vi "M686_scanning.vi"(5 "notifier out":refnum<notifier>, 6 "Velocity":dbl, 8 "Axis":bool[](array[boolean]), 9 "Positions":dbl[](array[numeric]), 10 "Action":T1=enum."MVR", 11 "VISA resource name":refnum<visa-resource-name>) -> (0 "Special Function":string, 1 "Status":bool, 2 "Position Out":dbl[](array[numeric]))   [LabVIEW 2011]
uses:
  Controls/StageStates.ctl
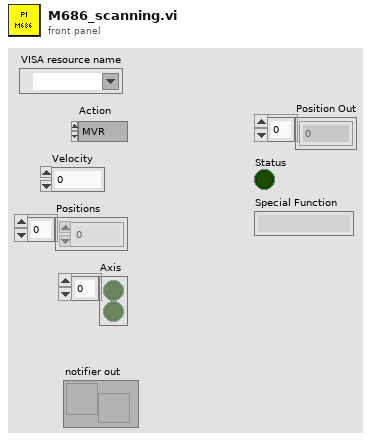
[diagram p1: front panel]
types:
  T1 = typedef "StageStates.ctl" = enum16{"POSITION", "MVR", "MOVE", "HALT", "ONTARGET", "ERROR", "EXIT", "HOME", "ZEROPOS", "NANOPOS", "QUIT", "ANALOG"}
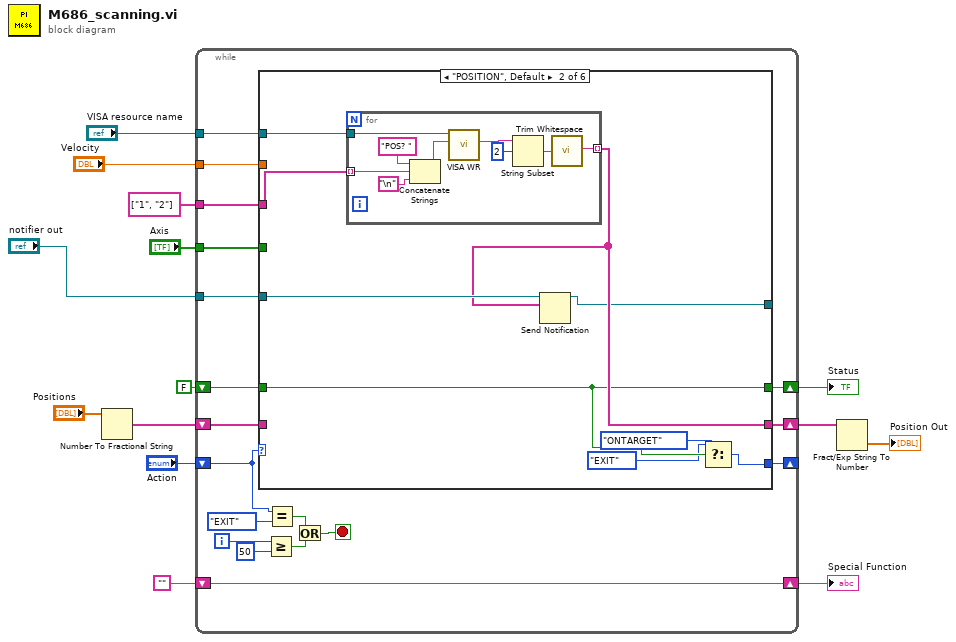
[diagram p0: block diagram]
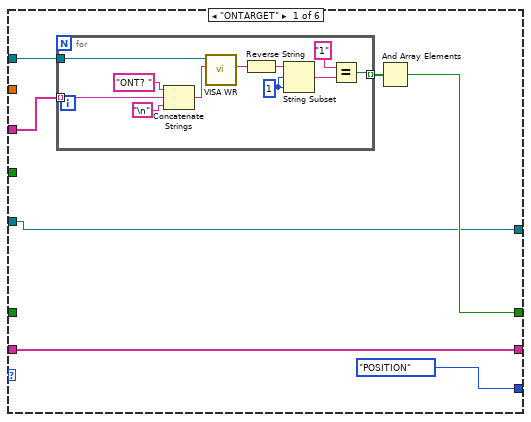
[diagram p2: hidden frame]
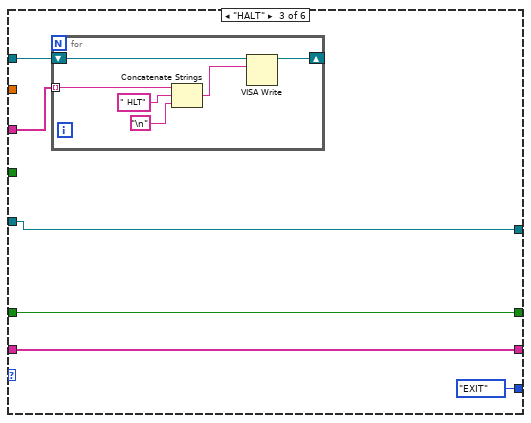
[diagram p3: hidden frame]
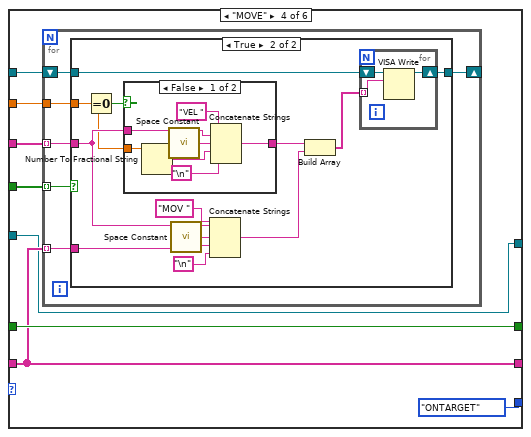
[diagram p4: hidden frame]
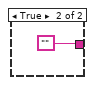
[diagram p6: hidden frame]
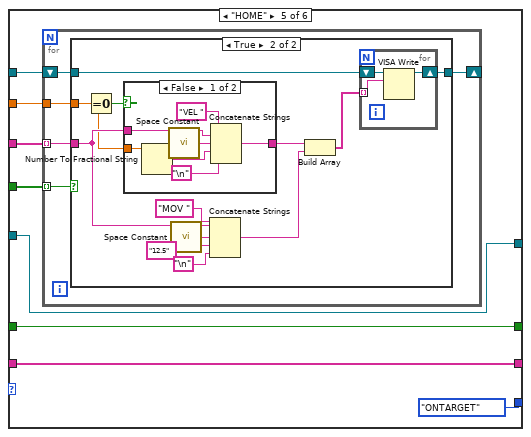
[diagram p7: hidden frame]
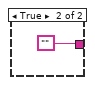
[diagram p9: hidden frame]
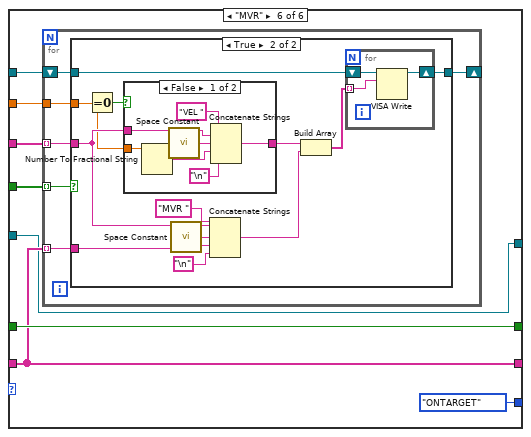
[diagram p10: hidden frame]
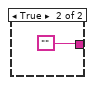
[diagram p12: hidden frame]
diagram:
  n1 = Number To Fractional String(number="Positions") -> (F-format string=w6:string[])  [unwired: 3 in]
  n2 = while {
    tunnel: string[] ["1", "2"] -> [w32]
    tunnel: "VISA resource name" -> [w31]
    shift-right: [w16] -> _
    shift-left: "Action" -> [w26]
    shift-right: [w29] -> w4
    shift-left: w6 -> [w30]
    shift-right: [w27] -> w11
    shift-left: FALSE -> [w28]
    tunnel: "Axis" -> [w20]
    tunnel: "Velocity" -> [w19]
    shift-right: [w18] -> w7
    shift-left: "" -> [w18]
    tunnel: "notifier out" -> [w15]
    i -> [w24]
    stop <- w22 stop-if-true
    n3 = case shown="\"POSITION\", Default" w26 {
      tunnel: w32 -> [w35 w58 w74 w88 w126 w163]
      tunnel: w31 -> [w39 w59 w73 w87 w125 w162]
      tunnel: w30 -> [w37 _ w72 w85 w123 w160]
      tunnel: [w37 w56 w72 w85 w123 w160] -> w29
      tunnel: w28 -> [_ w54 w71 w86 w124 w161]
      tunnel: [w36 w54 w71 w86 w124 w161] -> w27
      tunnel: w20 -> [_ _ _ w84 w122 w159]
      tunnel: w19 -> [_ _ _ w83 w121 w158]
      tunnel: [StageStates."POSITION" ("Action") w51 StageStates."EXIT" ("Action") StageStates."ONTARGET" ("Action") StageStates."ONTARGET" ("Action") StageStates."ONTARGET" ("Action")] -> w16
      tunnel: w15 -> [w34 w57 w69 w81 w119 w156]
      tunnel: [w34 w55 w69 w81 w119 w156] -> _
      frame "ONTARGET" {
        n4 = for {
          tunnel: w39 -> [w50]
          tunnel: [w45] -> w38 mode=indexing
          tunnel: w35 -> [w40] mode=indexing
          w41 = 1 ("length (rest)")
          n5 = Concatenate Strings("ONT? " ("string"), w40, "\n") -> (w49:string)
          n6 = call "VISA WR.vi"("write buffer"=w49, "VISA Refnum in"=w50) -> ("read buffer"=w48:string)  [unwired: 7 in, 2 out]
          n7 = Reverse String(1:w48) -> (0:w42:string)
          n8 = String Subset(string=w42, offset (0)=w41, length (rest)=w41) -> (substring=w47:string)
          n9 = Equal?(x="1", y=w47) -> (x = y?=w45:bool)
        }
        n10 = And Array Elements(Boolean array=w38) -> (logical AND=w36:bool)
      }
      frame "POSITION", Default {
        n11 = for {
          tunnel: w59 -> [w68]
          tunnel: [w65] -> w56 mode=indexing
          tunnel: w58 -> [w60] mode=indexing
          n12 = Concatenate Strings("POS? " ("string"), w60, "\n") -> (w67:string)
          n13 = call "VISA WR.vi"("write buffer"=w67, "VISA Refnum in"=w68) -> ("read buffer"=w66:string)  [unwired: 7 in, 2 out]
          n14 = String Subset(string=w66, offset (0)=2) -> (substring=w61:string)  [unwired: 1 in]
          n15 = call <vilib>:"Trim Whitespace.vi"("string"=w61) -> ("trimmed string"=w65:string)  [unwired: 1 in]
        }
        n16 = Send Notification(notification=w56, notifier=w57) -> (notifier out=w55:refnum<notifier>)  [unwired: 1 in, 1 out]
        n17 = Select(t=StageStates."EXIT" ("Action"), s=w54, f=StageStates."ONTARGET") -> (s? t:f=w51:T1)
      }
      frame "HALT" {
        n18 = for {
          tunnel: w74 -> [w78] mode=indexing
          shift-right: [w75] -> _
          shift-left: w73 -> [w76]
          n19 = Concatenate Strings(w78, " HLT" ("string"), "\n") -> (w77:string)
          n20 = VISA Write(VISA resource name=w76, write buffer=w77) -> (VISA resource name out=w75:refnum<visa-resource-name>)  [unwired: 1 in, 2 out]
        }
      }
      frame "MOVE" {
        n21 = for {
          tunnel: w88 -> [w94] mode=indexing
          tunnel: w85 -> [w93] mode=indexing
          shift-right: [w91] -> _
          shift-left: w87 -> [w92]
          tunnel: w84 -> [w90] mode=indexing
          tunnel: w83 -> [w89]
          n22 = case shown="True" w90 {
            tunnel: w94 -> [_ w101]
            tunnel: w93 -> [_ w104]
            tunnel: w92 -> [w95 w103]
            tunnel: [w95 w102] -> w91
            tunnel: w89 -> [_ w100]
            frame False {
            }
            frame True {
              n23 = Equal To 0?(x=w100) -> (x = 0?=w99:bool)
              n24 = case shown="False" w99 {
                tunnel: w101 -> [w114 _]
                tunnel: w100 -> [w111 _]
                tunnel: [w113 ""] -> w98
                frame False {
                  n25 = Number To Fractional String(number=w111) -> (F-format string=w112:string)  [unwired: 3 in]
                  n26 = call <vilib>:"Space Constant.vi"() -> ("String"=w117:string)
                  n27 = Concatenate Strings("VEL ", w114, w117, w112, "\n") -> (w113:string)
                }
                frame True {
                }
              }
              n28 = call <vilib>:"Space Constant.vi"() -> ("String"=w105:string)
              n29 = Concatenate Strings("MOV ", w101, w105, w104, "\n") -> (w97:string)
              n30 = Build Array(w98, w97) -> (w96:string[])
              n31 = for {
                shift-right: [w109] -> w102
                shift-left: w103 -> [w110]
                tunnel: w96 -> [w108] mode=indexing
                n32 = VISA Write(VISA resource name=w110, write buffer=w108) -> (VISA resource name out=w109:refnum<visa-resource-name>)  [unwired: 1 in, 2 out]
              }
            }
          }
        }
      }
      frame "HOME" {
        n33 = for {
          tunnel: w126 -> [w131] mode=indexing
          shift-right: [w129] -> _
          shift-left: w125 -> [w130]
          tunnel: w122 -> [w128] mode=indexing
          tunnel: w121 -> [w127]
          n34 = case shown="True" w128 {
            tunnel: w131 -> [_ w139]
            tunnel: w130 -> [w132 w141]
            tunnel: [w132 w140] -> w129
            tunnel: w127 -> [_ w138]
            frame False {
            }
            frame True {
              n35 = Equal To 0?(x=w138) -> (x = 0?=w137:bool)
              n36 = case shown="False" w137 {
                tunnel: w139 -> [w151 _]
                tunnel: w138 -> [w148 _]
                tunnel: [w150 ""] -> w136
                frame False {
                  n37 = Number To Fractional String(number=w148) -> (F-format string=w149:string)  [unwired: 3 in]
                  n38 = call <vilib>:"Space Constant.vi"() -> ("String"=w154:string)
                  n39 = Concatenate Strings("VEL ", w151, w154, w149, "\n") -> (w150:string)
                }
                frame True {
                }
              }
              n40 = call <vilib>:"Space Constant.vi"() -> ("String"=w142:string)
              n41 = Concatenate Strings("MOV ", w139, w142, "12.5" ("string"), "\n") -> (w135:string)
              n42 = Build Array(w136, w135) -> (w134:string[])
              n43 = for {
                shift-right: [w146] -> w140
                shift-left: w141 -> [w147]
                tunnel: w134 -> [w145] mode=indexing
                n44 = VISA Write(VISA resource name=w147, write buffer=w145) -> (VISA resource name out=w146:refnum<visa-resource-name>)  [unwired: 1 in, 2 out]
              }
            }
          }
        }
      }
      frame "MVR" {
        n45 = for {
          tunnel: w163 -> [w169] mode=indexing
          tunnel: w160 -> [w168] mode=indexing
          shift-right: [w166] -> _
          shift-left: w162 -> [w167]
          tunnel: w159 -> [w165] mode=indexing
          tunnel: w158 -> [w164]
          n46 = case shown="True" w165 {
            tunnel: w169 -> [_ w176]
            tunnel: w168 -> [_ w179]
            tunnel: w167 -> [w170 w178]
            tunnel: [w170 w177] -> w166
            tunnel: w164 -> [_ w175]
            frame False {
            }
            frame True {
              n47 = Equal To 0?(x=w175) -> (x = 0?=w174:bool)
              n48 = case shown="False" w174 {
                tunnel: w176 -> [w189 _]
                tunnel: w175 -> [w187 _]
                tunnel: [w188 ""] -> w173
                frame False {
                  n49 = Number To Fractional String(number=w187) -> (F-format string=w186:string)  [unwired: 3 in]
                  n50 = call <vilib>:"Space Constant.vi"() -> ("String"=w192:string)
                  n51 = Concatenate Strings("VEL ", w189, w192, w186, "\n") -> (w188:string)
                }
                frame True {
                }
              }
              n52 = call <vilib>:"Space Constant.vi"() -> ("String"=w180:string)
              n53 = Concatenate Strings("MVR ", w176, w180, w179, "\n") -> (w172:string)
              n54 = Build Array(w173, w172) -> (w171:string[])
              n55 = for {
                shift-right: [w184] -> w177
                shift-left: w178 -> [w185]
                tunnel: w171 -> [w183] mode=indexing
                n56 = VISA Write(VISA resource name=w185, write buffer=w183) -> (VISA resource name out=w184:refnum<visa-resource-name>)  [unwired: 1 in, 2 out]
              }
            }
          }
        }
      }
    }
    n57 = Greater Or Equal?(x=w24, y=50) -> (x >= y?=w21:bool)
    n58 = Equal?(x=w26, y=StageStates."EXIT") -> (x = y?=w25:bool)
    n59 = Or(x=w25, y=w21) -> (x .or. y?=w22:bool)
  }
  "Status" <- w11
  "Special Function" <- w7
  n60 = Fract/Exp String To Number(string=w4) -> (number=→"Position Out":dbl[])  [unwired: 3 in, 1 out]
